vi "Get Input DMA Refs.vi"(8 "error in (no error)":errorcluster, 9 "FPGA Ref":refnum<k20>, 10 "Item GUID":string, 11 "Section Ref in":T7 format="%.0x") -> (0 "error out":errorcluster, 1 "FPGA Ref":refnum<k20>, 2 "DMA Settings":T1[](array[typedef]) {"Write to VS Engine"."Pairs"."Refs" format="%.0x"; "DMA Settings"."dt" format="%#_p"; "DMA Settings"."Update Rate" items=["1 Hz"=1, "2 Hz"=2, "5 Hz"=5, "10 Hz"=10]}, 3 "Section Ref out":T7 format="%.0x")   [LabVIEW 2013, in "FPGA Addon Engine.lvlib"]
uses:
  FPGA Addon Engine.lvlib
  <vilib>/NI Veristand/Custom Device API/Custom Device Item Ref.ctl
  Types/DMA Input Settings.ctl
  <vilib>/NI VeriStand/Custom Device Waveform API/Multiple Waveforms Write (DBL)/Multiple Waveforms Write (DBL).lvclass
  Shared/DMA Settings.ctl
  Shared/Delacing Scheme.ctl
  Types/DMA Input Ref.ctl
  Inline Async API/Controls/Write To VS Engine.ctl
  <vilib>/NI Veristand/Custom Device API/Data Reference.ctl
  Shared/FG Action.ctl
  <vilib>/NI/LVFPGA Adv Session Resources/OpenByNameSubVI.vi
  <vilib>/rvi/interface/common/niFpgaWaitOnOcc.vi
  <vilib>/NI Veristand/Custom Device Tools/Custom Device Utility Library/NI VeriStand - Search for Item by GUID.vi
  Shared/Constants.vi
  <vilib>/NI Veristand/Custom Device API/Get Item Property (Variant).vi
  <vilib>/NI Veristand/Custom Device Waveform API/Multiple Waveforms Write (DBL)/NI VeriStand - Open Multiple Waveforms Write Session (DBL).vi
  <vilib>/NI Veristand/Custom Device Tools/Custom Device Utility Library/NI VeriStand - Search for All Items by GUID.vi
  <vilib>/NI Veristand/Custom Device API/Get Item Property (String).vi
  <vilib>/rvi/interface/common/dynamic/niFpgaEscapeDelimiterAndNull.vi
  <vilib>/Utility/error.llb/Error Cluster From Error Code.vi
  <vilib>/NI/LVFPGA Adv Session Resources/OpenByName.xnode
  <vilib>/rvi/interface/nirviMethod/nirviMethod.xnode
  Shared/FPGA Addon Shared.lvlib
  <vilib>/NI VeriStand/Custom Device API/Custom Device API.lvlib
  <vilib>/NI Veristand/Custom Device Tools/Custom Device Utility Library/Custom Device Utility Library.lvlib
  <vilib>/NI VeriStand/Custom Device Waveform API/NI_VS Custom Device Waveform API.lvlib
  <vilib>/rvi/errors/niLvFpgaMergeErrorWithErrorCode.vi
  Inline Async API/Inline Async API.lvlib
  <vilib>/FPGAPlugInAG/Dynamic/niLvFpga_StartFifo_Dynamic.vi
  <vilib>/NI/LVFPGA Adv Session Resources/LVFPGAAdvSessionResources.lvlib
  <vilib>/FPGAPlugInAG/Dynamic/niLvFpga_ConfigureFifo_Dynamic.vi
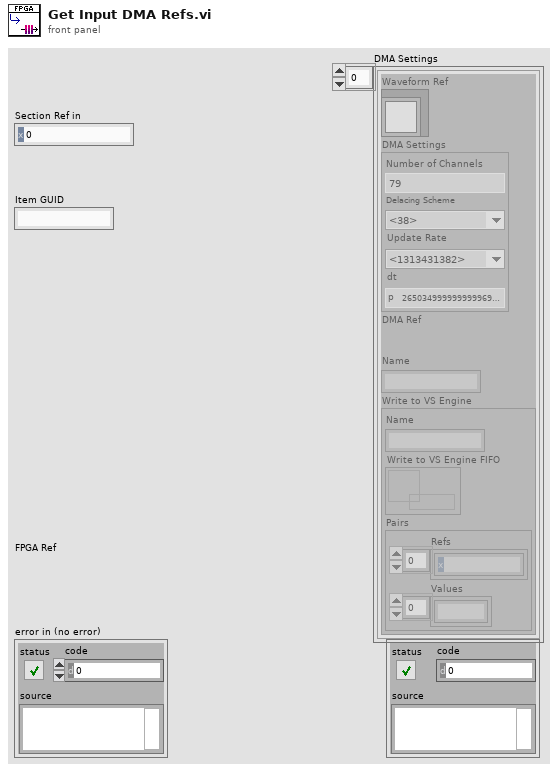
[diagram p1: front panel]
types:
  T1 = typedef "FPGA Addon Engine.lvlib/DMA Input Settings.ctl" = cluster{"Waveform Ref":refnum<class "Multiple Waveforms Write (DBL).lvclass">, "DMA Settings":T2, "DMA Ref":T4, "Name":string, "Write to VS Engine":T5}
  T2 = typedef "FPGA Addon Shared.lvlib/DMA Settings.ctl" = cluster{"Number of Channels":u8, "Delacing Scheme":T3, "Update Rate":u32, "dt":dbl}
  T3 = typedef "FPGA Addon Shared.lvlib/Delacing Scheme.ctl" = enum8{"Interlaced"}
  T4 = typedef "FPGA Addon Engine.lvlib/DMA Input Ref.ctl" = refnum<k20>
  T5 = typedef "FPGA Addon Engine.lvlib/Inline Async API.lvlib/Write To VS Engine.ctl" = cluster{"Name":string, "Write to VS Engine FIFO":refnum<k33>, "Pairs":cluster{"Refs":T6[], "Values":dbl[]}}
  T6 = typedef "Custom Device API.lvlib/Data Reference.ctl" = i32
  T7 = typedef "Custom Device API.lvlib/Custom Device Item Ref.ctl" = u64
  T8 = typedef "FPGA Addon Shared.lvlib/FG Action.ctl" = enum8{"GET", "SET"}
  T9 = typedef "Fifo_DMA_Config.ctl" = cluster{"Name":string, "Depth":u32, "Write? (Deprecated:Use Implementation)":bool, "Physical Channel":u32, "Base Address":u32, "Data Width":u32, "Data Type":T10, "FXP Properties":variant, "Write Window Address":u32, "Implementation":T11, "Control Set":u32}
  T10 = typedef "niFpgaDataTypeControl.ctl" = enum32{"Boolean", "I8", "I16", "I32", "I64", "U8", "U16", "U32", "U64", "FXP", "CustomControl", "SGL"}
  T11 = typedef "niFpgaDmaChannelImplementation.ctl" = enum16{"niFpgaTargetToHost", "niFpgaHostToTarget", "niFpgaPeerToPeerWriter", "niFpgaPeerToPeerReader", "niCoreTargetToHost", "niCoreHostToTarget"}
  T12 = cluster{"Name":string, "Depth":u32, "Write? (Deprecated:Use Implementation)":bool, "Physical Channel":u32, "Base Address":u32, "Data Width":u32, "Data Type":enum32{"Boolean", "I8", "I16", "I32", "I64", "U8", "U16", "U32", "U64", "FXP", "CustomControl", "SGL"}, "FXP Properties":variant, "Write Window Address":u32, "Implementation":enum16{"niFpgaTargetToHost", "niFpgaHostToTarget", "niFpgaPeerToPeerWriter", "niFpgaPeerToPeerReader", "niCoreTargetToHost", "niCoreHostToTarget"}, "Control Set":u32}[]
  T13 = cluster{"Name":string, "type":variant, "indicator?":bool}[]
  T14 = typedef "Custom Device API.lvlib/Waveform Data Reference.ctl" = i32
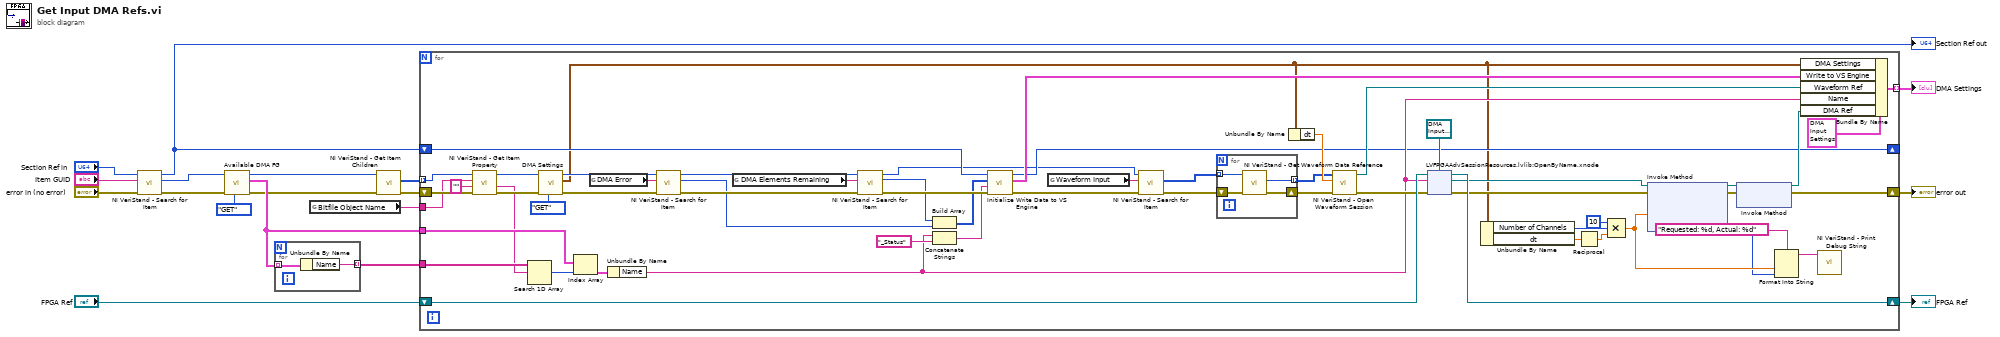
[diagram p0: block diagram]
diagram:
  n1 = call-poly <vilib>:"NI VeriStand - Search for Item.vi"("error in"="error in (no error)", "Item GUID"="Item GUID", "Section Ref in"="Section Ref in") -> ("error out"=w15:errorcluster, "Item Ref"=w17:T7, "Section Ref out"=w1:T7)  [unwired: 5 in, 1 out]
  "Section Ref out" <- w1
  n2 = call "Available DMA FG.vi"("Action"=FG_Action."GET", "error in (no error)"=w15, "Item Ref"=w17) -> ("error out"=w11:errorcluster, "Available DMA"=w12:T9[], "Item Ref out"=w13:T7)  [unwired: 6 in]
  n3 = for {
    tunnel: w12 -> [w20] mode=indexing
    tunnel: [w19] -> w10 mode=indexing
    n4 = Unbundle By Name(w20) -> ("Name"=w19:string)
  }
  n5 = global read "Constants.vi" "Bitfile Object Name"() -> (w9:string)
  n6 = call <vilib>:"NI VeriStand - Get Item Children.vi"("error in (no error)"=w11, "Item Ref in"=w13) -> ("error out"=w7:errorcluster, "Child Refs"=w8:T7[])  [unwired: 6 in, 2 out]
  n7 = for {
    shift-right: [w50] -> w3
    shift-left: w7 -> [w78]
    tunnel: w8 -> [w77] mode=indexing
    tunnel: w9 -> [w76]
    tunnel: w10 -> [w74]
    tunnel: w12 -> [w73]
    shift-right: [w67] -> w4
    shift-left: "FPGA Ref" -> [w68]
    tunnel: [w65] -> w2 mode=indexing
    shift-right: [w27] -> _
    shift-left: w1 -> [w28]
    n8 = call-poly <vilib>:"NI VeriStand - Get Item Property.vi"("error in (no error)"=w78, "Default Value"="", "Property Name"=w76, "Item Ref in"=w77) -> ("error out"=w64:errorcluster, "Value"=w54:string, "Item Ref out"=w63:T7)  [unwired: 4 in, 1 out]
    n9 = Search 1D Array(1D array=w74, element=w54) -> (index of element=w72:i32)  [unwired: 1 in]
    n10 = call "DMA Settings.vi"("Action"=FG_Action."GET", "error in (no error)"=w64, "Item Ref"=w63) -> ("error out"=w42:errorcluster, "DMA Settings"=w25:T2, "Item Ref out"=w41:T7)  [unwired: 6 in]
    n11 = Index Array(array=w73, index=w72) -> (element=w70:T9)
    n12 = global read "Constants.vi" "DMA Error"() -> (w43:string)
    n13 = Unbundle By Name(w70) -> ("Name"=w31:string)
    n14 = call-poly <vilib>:"NI VeriStand - Search for Item.vi"("error in"=w42, "Item GUID"=w43, "Section Ref in"=w41) -> ("error out"=w39:errorcluster, "Item Ref"=w35:T7, "Section Ref out"=w38:T7)  [unwired: 5 in, 1 out]
    n15 = global read "Constants.vi" "DMA Elements Remaining"() -> (w40:string)
    n16 = call-poly <vilib>:"NI VeriStand - Search for Item.vi"("error in"=w39, "Item GUID"=w40, "Section Ref in"=w38) -> ("error out"=w37:errorcluster, "Item Ref"=w34:T7, "Section Ref out"=w26:T7)  [unwired: 5 in, 1 out]
    n17 = Build Array(w34, w35) -> (w33:T7[])
    n18 = Concatenate Strings(w31, "_Status" ("FIFO Name")) -> (w30:string)
    n19 = call "Initialize Write Data to VS Engine.vi"("error in (no error)"=w37, "FIFO Name"=w30, "Hardware Output Refs"=w33, "Device Ref"=w28) -> ("error out"=w36:errorcluster, "Write to VS Engine"=w29:T5, "Device Ref out"=w27:T7)  [unwired: 5 in]
    n20 = global read "Constants.vi" "Waveform Input"() -> (w55:string)
    n21 = call-poly <vilib>:"NI VeriStand - Search for Item.vi"("error in"=w36, "Item GUID"=w55, "Section Ref in"=w26) -> ("error out"=w57:errorcluster, "Item Refs"=w56:T7[])  [unwired: 5 in, 2 out]
    n22 = for {
      tunnel: w56 -> [w82] mode=indexing
      tunnel: [w81] -> w59 mode=indexing
      shift-right: [w79] -> w58
      shift-left: w57 -> [w80]
      n23 = call <vilib>:"NI VeriStand - Get Waveform Data Reference.vi"("error in (no error)"=w80, "Waveform Ref in"=w82) -> ("error out"=w79:errorcluster, "Waveform Data Reference"=w81:T14)  [unwired: 7 in, 1 out]
    }
    n24 = Unbundle By Name(w25) -> ("dt"=w60:dbl)
    n25 = call-poly <vilib>:"NI VeriStand - Open Waveform Session.vi"("error in (no error)"=w58, "dt"=w60, "DBL Waveform Data References"=w59) -> ("error out"=w61:errorcluster, "Multiple Waveforms Write Session (DBL)"=w62:refnum<class "Multiple Waveforms Write (DBL).lvclass">)  [unwired: 7 in]
    n26 = xnode "LVFPGAAdvSessionResources.lvlib:OpenByName.xnode"("FPGA VI Reference in"=w68, "Resource name in"=w31, "Single resource reference type in"=T4 refnum, "Error in"=w61) -> ("Single resource reference out"=w49:T4, "Error out"=w51:errorcluster, "FPGA VI Reference out"=w67:refnum<k20>)
    n27 = Unbundle By Name(w25) -> ("Number of Channels"=w45:u8, "dt"=w47:dbl)
    n28 = Reciprocal(x=w47) -> (1/x=w46:dbl)
    n29 = Compound Arithmetic op=MULTIPLY(u8 10 ("value"), w45, w46) -> (w24:dbl)
    n30 = xnode "Invoke Method"("FPGA VI Reference In"=w49, "error in"=w51, "Requested Depth"=w24) -> ("FPGA VI Reference Out"=w53:T4, "error out"=w52:errorcluster, "Actual Depth"=w23:u32)
    n31 = xnode "Invoke Method"("FPGA VI Reference In"=w53, "error in"=w52) -> ("FPGA VI Reference Out"=w48:T4, "error out"=w50:errorcluster)
    n32 = Format Into String(format string="Requested: %d, Actual: %d", w24, w23) -> (resulting string=w21:string)  [unwired: 2 in, 1 out]
    n33 = Bundle By Name(cluster=T1 {"Waveform Ref"=refnum, "DMA Settings"={"Number of Channels"=0, "Delacing Scheme"=enum."Interlaced", "Update Rate"=0, "dt"=0.0}, "DMA Ref"=refnum, "Name"="", "Write to VS Engine"={"Name"="", "Write to VS Engine FIFO"=refnum, "Pairs"={"Refs"=[], "Values"=[]}}}, "DMA Settings"=w25, "Write to VS Engine"=w29, "Waveform Ref"=w62, "Name"=w31, "DMA Ref"=w48) -> (w65:T1)
    n34 = call <vilib>:"NI VeriStand - Print Debug String.vi"("Message"=w21) -> ()  [unwired: 10 in, 1 out]
  }
  "error out" <- w3
  "FPGA Ref" <- w4
  "DMA Settings" <- w2
